vi "Open Application.vi"(4 "enable interaction (false)":bool, 6 "visible (false)":bool=TRUE, 8 "error in (no error)":errorcluster) -> (0 "error out":errorcluster, 3 "JMP application":refnum<k7>)   [LabVIEW 2019, in "JMP Automation.lvlib"]
doc: "Get an handle to the JMP application. If JMP is closed, open it.\n\nvisible (false): if true show the JMP windows (can slow down the operations)\nenable interaction (false): if true display information in message boxes during an automated process rather than in the log. This option effectively turns off the Batch mode processing."
uses:
  <instrlib>/LV_JMP_bridge/JMP Automation.lvlib
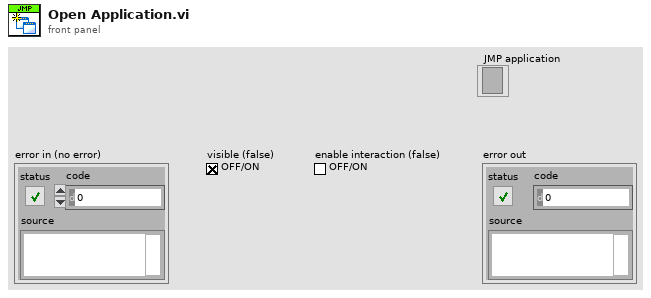
[diagram p1: front panel]
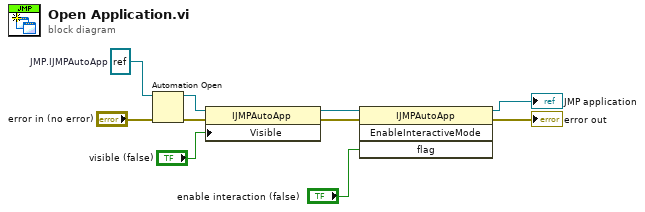
[diagram p0: block diagram]
diagram:
  w5 = refnum<k7> refnum  # JMP.IJMPAutoApp
  n1 = Automation Open(error in (no error)="error in (no error)", Automation Refnum=w5) -> (Automation Refnum=w6:refnum<k7>, error out=w7:errorcluster)  [unwired: 2 out]
  n2 = property class="IJMPAutoApp"(reference=w6, error in=w7, "Visible"="visible (false)") -> (reference out=w3:refnum<k7>, error out=w10:errorcluster)
  n3 = invoke class="IJMPAutoApp" method="EnableInteractiveMode"(reference=w3, error in=w10, "flag"="enable interaction (false)") -> (reference out=→"JMP application":refnum<k7>, error out=→"error out":errorcluster)  [unwired: 1 in, 2 out]
